vi "Init.vi"(8 "error in (no error)":errorcluster, 11 "Strings And Values []":T1) -> (0 "error out":errorcluster, 3 "Predefined Values out":refnum<class "Predefined Values.lvclass">)   [LabVIEW 2020, in "Dynamic Combobox.lvlib" / "Predefined Values.lvclass"]
uses:
  Predefined Values.lvclass
  Predefined Values.lvclass/Predefined Values.ctl
  <vilib>/Utility/miscctls.llb/LVComboBoxStrsAndValuesArrayTypeDef.ctl
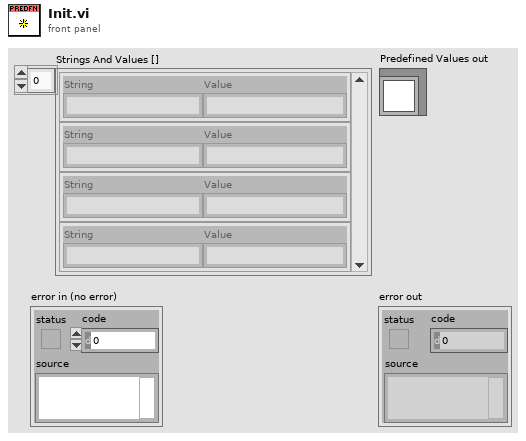
[diagram p1: front panel]
types:
  T1 = typedef "LVComboBoxStrsAndValuesArrayTypeDef.ctl" = cluster{"String":string, "Value":string}[]
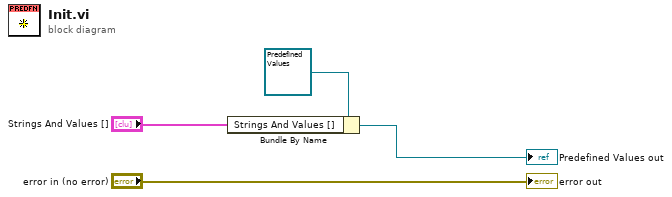
[diagram p0: block diagram]
diagram:
  n1 = Bundle By Name(cluster=refnum<class "Predefined Values.lvclass"> refnum ("Predefined Values in"), "Strings And Values []"="Strings And Values []") -> (→"Predefined Values out":refnum<class "Predefined Values.lvclass">)
  "error out" <- "error in (no error)"
